vi "test.vi"() -> ()   [LabVIEW 2013]
panel:
  in  "stop":bool
  out "Real 2":dbl
  in  "Real":dbl
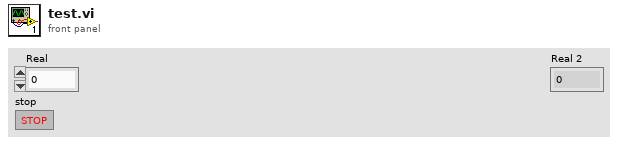
[diagram p1: front panel]
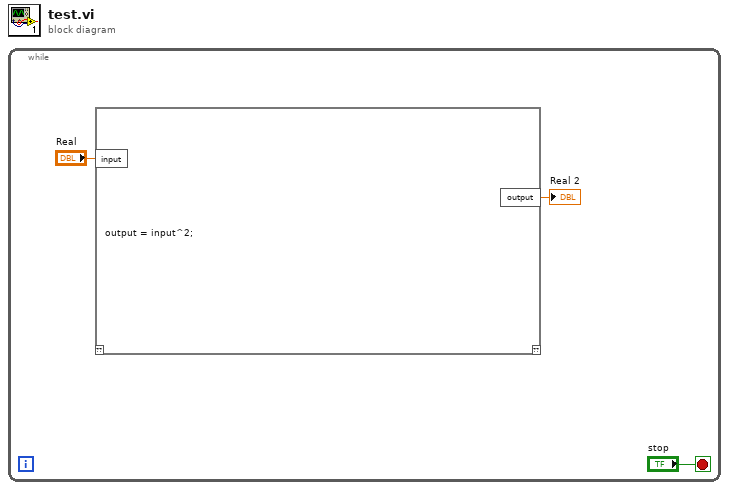
[diagram p0: block diagram]
diagram:
  n1 = while {
    stop <- "stop" stop-if-true
    n2 = script code="output = input^2;"("input"="Real") -> ("output"=→"Real 2":dbl)  [unwired: 1 in, 1 out]
  }
